vi "Generate_SDA_SCL.vi"() -> ()   [LabVIEW 2023]
panel:
  out "Waveform Graph":waveform(dbl)[](graph)
  in  "8Bit_Binary":bool[](array[boolean])
  in  "T_HD_DAT (uS)":dbl
  in  "T_Off (uS)":dbl
  in  "T_On (uS)":dbl
  in  "Frequency (kHz)":dbl
  in  "T_SU_DAT (uS)":dbl
  in  "T_HD_STA (uS)":i32
  in  "Off_Set (uS)":i32
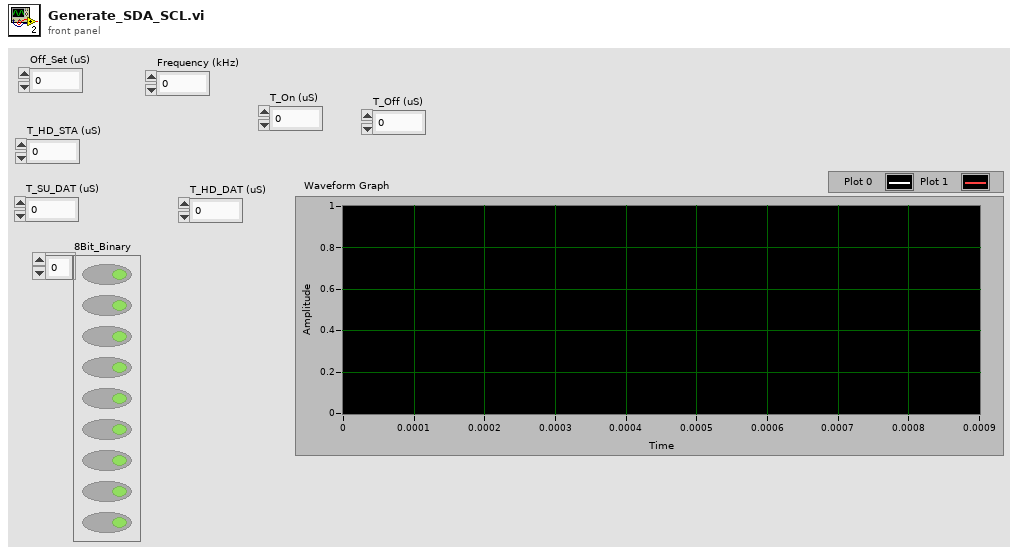
[diagram p1: front panel]
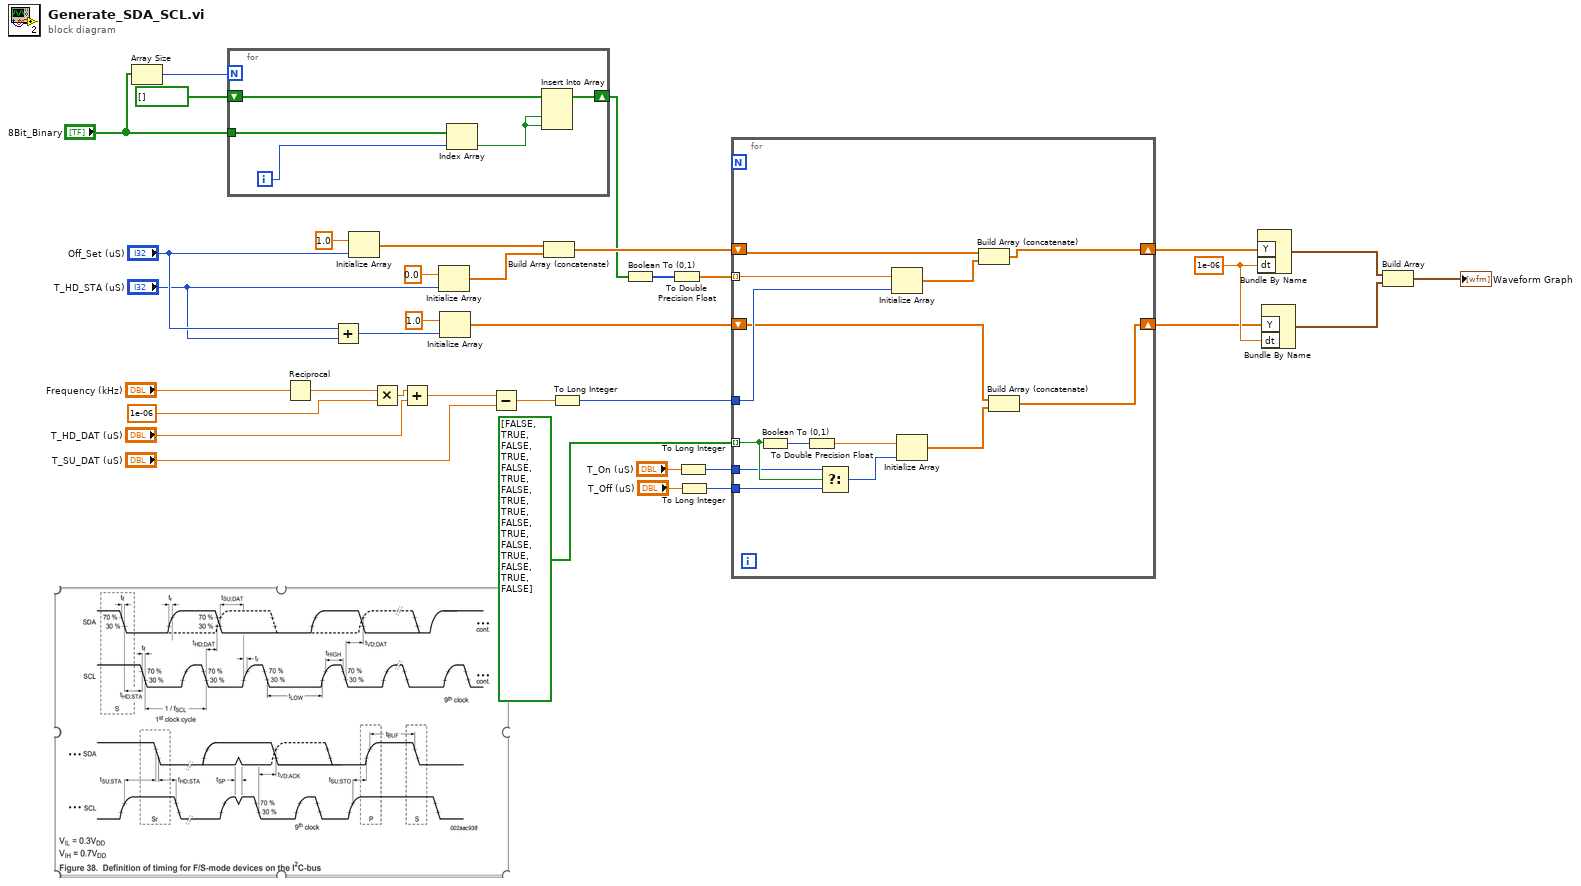
[diagram p0: block diagram]
diagram:
  w10 = 1e-06 ("dt")
  n1 = Array Size(array="8Bit_Binary") -> (size(s)=w2:i32)
  n2 = for {
    N: w2 -> [_]
    shift-right: [w38] -> w3
    shift-left: bool[] [] -> [w39]
    tunnel: "8Bit_Binary" -> [w37]
    i -> [w41]
    n3 = Index Array(array=w37, index=w41) -> (element=w40:bool)
    n4 = Insert Into Array(array=w39, new element #1=w40, new element #2=w40) -> (w38:bool[])  [unwired: 1 in]
  }
  n5 = Reciprocal(x="Frequency (kHz)") -> (1/x=w12:dbl)
  n6 = Add(x="Off_Set (uS)", y="T_HD_STA (uS)") -> (x+y=w29:i32)
  n7 = Initialize Array(1.0 ("element"), "Off_Set (uS)") -> (w34:dbl[])
  n8 = Multiply(x=w12, y=1e-06 ("dt")) -> (x*y=w13:dbl)
  n9 = Add(x=w13, y="T_HD_DAT (uS)") -> (x+y=w25:dbl)
  n10 = Initialize Array(0.0 ("element"), "T_HD_STA (uS)") -> (w33:dbl[])
  n11 = Initialize Array(1.0 ("element"), w29) -> (w28:dbl[])
  n12 = Subtract(x=w25, y="T_SU_DAT (uS)") -> (x-y=w23:dbl)
  n13 = Build Array (concatenate)(w34, w33) -> (w32:dbl[])
  n14 = To Long Integer(number=w23) -> (32bit integer=w20:i32)
  n15 = Boolean To (0,1)(Boolean=w3) -> (0, 1=w22:i16[])
  n16 = To Double Precision Float(number=w22) -> (double precision float=w21:dbl[])
  n17 = To Long Integer(number="T_On (uS)") -> (32bit integer=w16:i32)
  n18 = To Long Integer(number="T_Off (uS)") -> (32bit integer=w15:i32)
  n19 = for {
    shift-right: [w42] -> w9
    shift-left: w28 -> [w45]
    shift-right: [w43] -> w5
    shift-left: w32 -> [w55]
    tunnel: w21 -> [w53] mode=indexing
    tunnel: w20 -> [w52]
    tunnel: bool[] [FALSE, TRUE, FALSE, TRUE, FALSE, TRUE, FALSE, TRUE, TRUE, FALSE, TRUE, FALSE, TRUE, FALSE, TRUE, FALSE] ("8Bit_Binary") -> [w49] mode=indexing
    tunnel: w15 -> [w48]
    tunnel: w16 -> [w47]
    n20 = Boolean To (0,1)(Boolean=w49) -> (0, 1=w51:i16)
    n21 = To Double Precision Float(number=w51) -> (double precision float=w50:dbl)
    n22 = Select(t=w47, s=w49, f=w48) -> (s? t:f=w46:i32)
    n23 = Initialize Array(w53, w52) -> (w54:dbl[])
    n24 = Initialize Array(w50, w46) -> (w44:dbl[])
    n25 = Build Array (concatenate)(w55, w54) -> (w43:dbl[])
    n26 = Build Array (concatenate)(w45, w44) -> (w42:dbl[])
  }
  n27 = Bundle By Name("Y"=w5, "dt"=w10) -> (w8:waveform(dbl))  [unwired: 1 in]
  n28 = Bundle By Name("Y"=w9, "dt"=w10) -> (w7:waveform(dbl))  [unwired: 1 in]
  n29 = Build Array(w8, w7) -> (→"Waveform Graph":waveform(dbl)[])
